vi "Generate dynamically called windows folder path.vi"(1 "name of dynamically called VI":string="Window-Internal error message.vi") -> (0 "Dynamically called VI path":path)   [LabVIEW 2017]
panel:
  out "Current VI's Path (+ Relative)":path
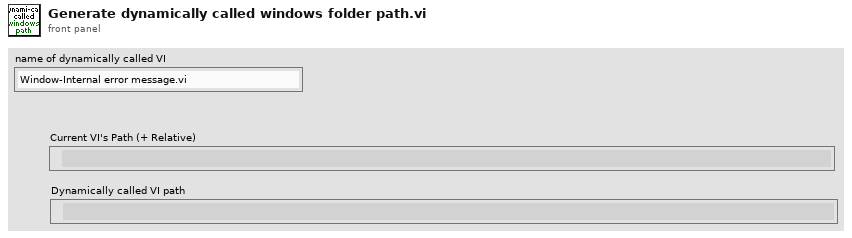
[diagram p1: front panel]
types:
  T1 = typedef "Fixed strings.ctl" = cluster{"ROI file name":string, "Normalised ROI file name":string, "Zplane Pockels values file name":string, "Functional data folder name":string, "Experiment Header file name":string, "Z-stack images folder name":string, "Groups setup rel. path":string, "Groups text file rel. path":string, "TDMS files folder name (F.img)":string, "TDMS files folder name (V.acq)":string, "TDMS files folder name (Pl.acq)":string, "Cycle rel times sequence file":string, "Dynamically called VIs folder name":string, "Time Series folder base name":string}
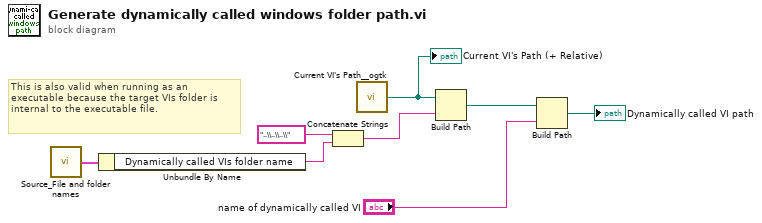
[diagram p0: block diagram]
diagram:
  # "This is also valid when running as an executable because the target VIs folder is internal to the executable file."
  n1 = call "Source_File and folder names.vi"() -> ("Fixed strings"=w1:T1)  [unwired: 1 in]
  n2 = Unbundle By Name(w1) -> ("Dynamically called VIs folder name"=w2:string)
  n3 = Concatenate Strings("..\\..\\..\\" ("VI Name"), w2) -> (w6:string)
  n4 = call <userlib>:"Current VI's Path__ogtk.vi"() -> ("Current VI's Path (+ Relative)"=w5:path)  [unwired: 1 in]
  "Current VI's Path (+ Relative)" <- w5
  n5 = Build Path(base path=w5, name or relative path=w6) -> (appended path=w8:path)
  n6 = Build Path(base path=w8, name or relative path="name of dynamically called VI") -> (appended path=→"Dynamically called VI path":path)
